vi "Z900_navX_Util_EncodeProtocol_Int8.vi"(1 "Int8":i8[](array[numeric])) -> (0 "Little Endian":u8[](array[numeric]))   [LabVIEW 2015, in "Apple Pi Gyro Library.lvlib" / "navX Library v2.lvlib"]
uses:
  navX Library v2.lvlib
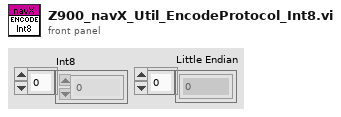
[diagram p1: front panel]
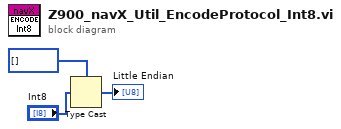
[diagram p0: block diagram]
diagram:
  n1 = Type Cast(type=u8[] [] ("Int8"), x="Int8") -> (*(type *) &x=→"Little Endian":u8[])
